vi "Siargo Get Total Flow.vi"(8 "error in (no error)":errorcluster, 11 "Modbus API in":refnum<class "Modbus API.lvclass">) -> (0 "error out":errorcluster, 2 "Totalized Flow (CuFt)":dbl format="%#.4g", 3 "Modbus API out":refnum<class "Modbus API.lvclass">)   [LabVIEW 2020]
uses:
  <vilib>/NI/Modbus Library/API/Modbus API.lvclass
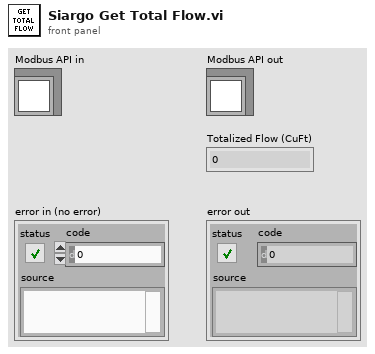
[diagram p1: front panel]
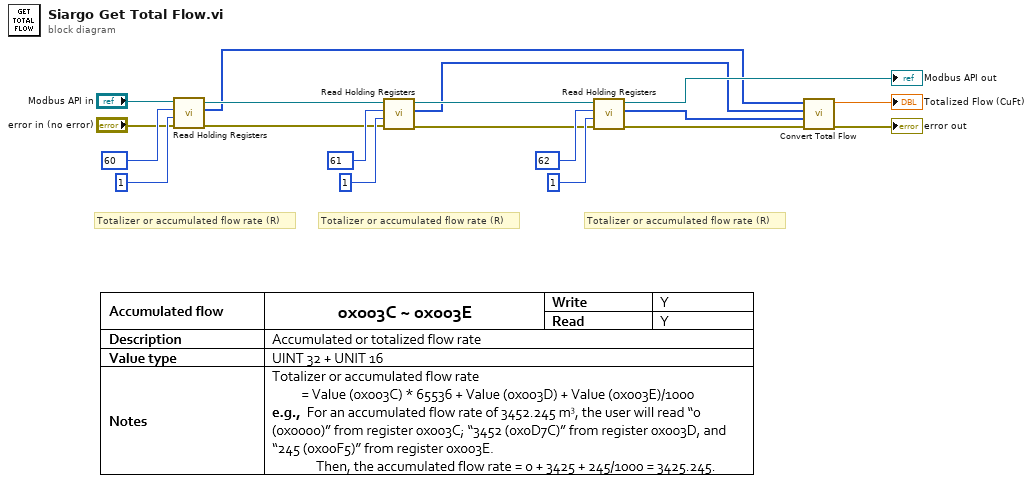
[diagram p0: block diagram]
diagram:
  # "Totalizer or accumulated flow rate (R)"
  # "Totalizer or accumulated flow rate (R)"
  # "Totalizer or accumulated flow rate (R)"
  n1 = call-dynamic "Read Holding Registers.vi"("error in"="error in (no error)", "number of inputs"=u16 1, "starting address"=u16 60, "Modbus instance in"="Modbus API in") -> ("error out"=w11:errorcluster, "register values"=w6:u16[], "Modbus instance out"=w7:refnum<class "Modbus API.lvclass">)  [unwired: 5 in]
  n2 = call-dynamic "Read Holding Registers.vi"("error in"=w11, "number of inputs"=u16 1, "starting address"=u16 61, "Modbus instance in"=w7) -> ("error out"=w10:errorcluster, "register values"=w5:u16[], "Modbus instance out"=w8:refnum<class "Modbus API.lvclass">)  [unwired: 5 in]
  n3 = call-dynamic "Read Holding Registers.vi"("error in"=w10, "number of inputs"=u16 1, "starting address"=u16 62, "Modbus instance in"=w8) -> ("error out"=w3:errorcluster, "register values"=w4:u16[], "Modbus instance out"=→"Modbus API out":refnum<class "Modbus API.lvclass">)  [unwired: 5 in]
  n4 = call "Convert Total Flow.vi"("error in (no error)"=w3, "3E"=w4, "3D"=w5, "3C"=w6) -> ("error out"=→"error out":errorcluster, "Totalized Flow (CuFt)"=→"Totalized Flow (CuFt)":dbl)  [unwired: 6 in]
